vi "Test Rotate String.vi"(8 "error in (no error)":errorcluster) -> (0 "error out":errorcluster, 3 "Pass?":bool)   [LabVIEW 2020]
uses:
  G-Unicode/Types/UTF-8 String/UTF-8 String.lvclass/UTF-8 String.ctl
  952276f3-5b34-4e34-8a1d-addec04de753.vi
  0ddb7cc8-26f8-44a6-9ae5-6ad694366a72.vi
  402b7c7c-7276-4835-8217-27b45ac813ca.vi
  G-Unicode/Private/Conversion/String as Encoded String.vi
  G-Unicode/Private/Conversion/Polymorphic VIs/String as Encoded String (LabVIEW String).vi
  G-Unicode/Private/Library/gu_rotate_string.vi
  G-Unicode/Private/Conversion/Polymorphic VIs/String as Encoded String (UTF-8 String).vi
  G-Unicode/Types/UTF-8 String/Read Encoded UTF-8 String.vi
  G-Unicode/Private/Library/gu_strlen.vi
  G-Unicode/Types/UTF-8 String/UTF-8 String.lvclass
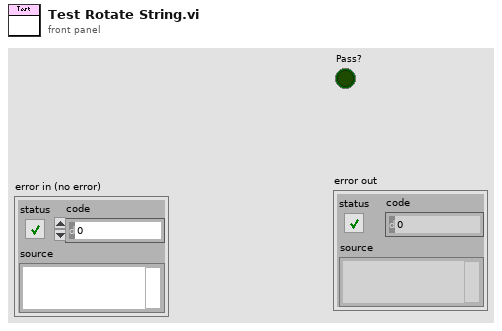
[diagram p1: front panel]
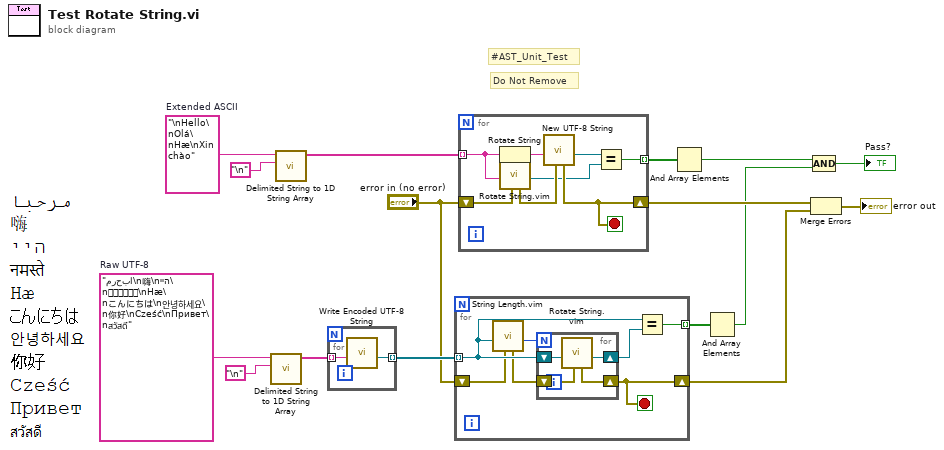
[diagram p0: block diagram]
diagram:
  w2 = "\nHello\nOlá\nHæ\nXin chào"  # Extended ASCII
  w15 = "مرحبا\n嗨\nהיי\nनमस्ते\nHæ\nこんにちは\n안녕하세요\n你好\nCześć\nПривет\nสวัสดี"  # Raw UTF-8
  # "Do Not Remove"
  # "#AST_Unit_Test"
  n1 = call <vilib>:"Delimited String to 1D String Array.vi"("delimiter"="\n", "delimited string"=w15) -> ("string array"=w14:string[])  [unwired: 9 in]
  n2 = call <vilib>:"Delimited String to 1D String Array.vi"("delimiter"="\n", "delimited string"=w2) -> ("string array"=w1:string[])  [unwired: 9 in]
  n3 = for {
    tunnel: w14 -> [w18] mode=indexing
    tunnel: [w17] -> w5 mode=indexing
    n4 = call "Write Encoded UTF-8 String.vi"("Encoded UTF-8 String"=w18) -> ("UTF-8 String"=w17:refnum<class "UTF-8 String.lvclass">)  [unwired: 10 in]
  }
  n5 = for {
    tunnel: w5 -> [w22] mode=indexing
    tunnel: [w25] -> w8 mode=indexing
    shift-right: [w23] -> w6
    shift-left: "error in (no error)" -> [w21]
    stop <- w23 stop-if-true
    n6 = call "String Length.vim"("error in"=w21, "String"=w22) -> ("Length"=w19:i32, "error out"=w20:errorcluster)  [unwired: 8 in]
    n7 = for {
      N: w19 -> [_]
      shift-right: [w28] -> w23
      shift-left: w20 -> [w29]
      shift-right: [w26] -> w24
      shift-left: w22 -> [w27]
      n8 = call "Rotate String.vim"("error in"=w29, "String"=w27) -> ("First Codepoint Last"=w26:refnum<class "UTF-8 String.lvclass">, "error out"=w28:errorcluster)  [unwired: 8 in]
    }
    n9 = Equal?(x=w22, y=w24) -> (x = y?=w25:bool)
  }
  n10 = for {
    tunnel: [w37] -> w10 mode=indexing
    shift-right: [w32] -> w13
    shift-left: "error in (no error)" -> [w35]
    tunnel: w1 -> [w36] mode=indexing
    stop <- w32 stop-if-true
    n11 = Rotate String(1:w36) -> (0:w34:string)
    n12 = call "Rotate String.vim"("error in"=w35, "String"=w36) -> ("First Codepoint Last"=w31:refnum<class "UTF-8 String.lvclass">, "error out"=w33:errorcluster)  [unwired: 8 in]
    n13 = call "New UTF-8 String.vi"("error in"=w33, "LabVIEW String"=w34) -> ("UTF-8 String"=w30:refnum<class "UTF-8 String.lvclass">, "error out"=w32:errorcluster)  [unwired: 8 in]
    n14 = Equal?(x=w30, y=w31) -> (x = y?=w37:bool)
  }
  n15 = And Array Elements(Boolean array=w10) -> (logical AND=w9:bool)
  n16 = And Array Elements(Boolean array=w8) -> (logical AND=w7:bool)
  n17 = Merge Errors(w13, w6) -> (→"error out":errorcluster)
  n18 = Compound Arithmetic op=AND(w9, w7) -> (→"Pass?":bool)
